vi "setAVGFilterStatus.vi"(8 "error in (no error)":errorcluster, 9 "Measurement Function (0: Current)":T2, 10 "AVG Filter type":T1, 11 "Electrometer in":refnum<class "Electrometer.lvclass">) -> (0 "error out":errorcluster, 3 "Electrometer out":refnum<class "Electrometer.lvclass">)   [LabVIEW 2016, in "Electrometer.lvclass"]
uses:
  Electrometer.lvclass
  Modes.ctl
  AVG Filter type.ctl
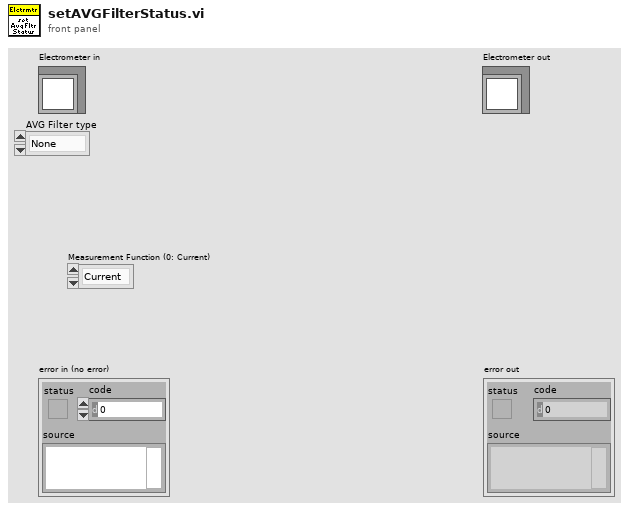
[diagram p1: front panel]
types:
  T1 = typedef "Electrometer.lvclass/AVG Filter type.ctl" = enum16{"None", "Scalar", "Advanced"}
  T2 = typedef "Electrometer.lvclass/Modes.ctl" = enum16{"Current", "Charge", "Voltage", "Resistance"}
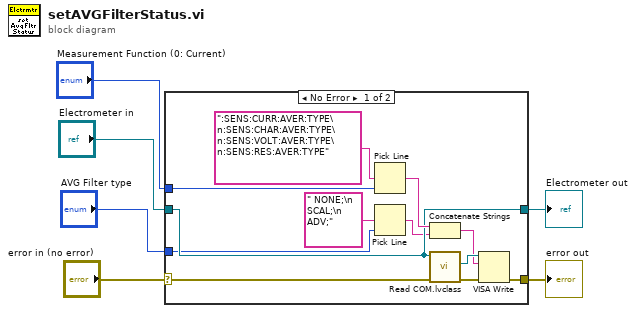
[diagram p0: block diagram]
diagram:
  n1 = case shown="No Error" "error in (no error)" {
    selector: "error in (no error)" -> [w13 w20]
    tunnel: [w11 w20] -> w5
    tunnel: [w14 w19] -> w3
    tunnel: "Electrometer in" -> [w14 w19]
    tunnel: "Measurement Function (0: Current)" -> [w10 _]
    tunnel: "AVG Filter type" -> [w7 _]
    frame No Error {
      n2 = Pick Line(multi-line string=":SENS:CURR:AVER:TYPE\n:SENS:CHAR:AVER:TYPE\n:SENS:VOLT:AVER:TYPE\n:SENS:RES:AVER:TYPE", line index=w10) -> (output string=w15:string)  [unwired: 1 in]
      n3 = Pick Line(multi-line string=" NONE;\n SCAL;\n ADV;", line index=w7) -> (output string=w8:string)  [unwired: 1 in]
      n4 = Concatenate Strings(w15, w8) -> (w17:string)
      n5 = call "Read COM.lvclass.vi"("error in (no error)"=w13, "Electrometer in"=w14) -> ("error out"=w12:errorcluster, "VISA"=w18:refnum<visa-resource-name>)  [unwired: 7 in, 1 out]
      n6 = VISA Write(VISA resource name=w18, write buffer=w17, error in (no error)=w12) -> (error out=w11:errorcluster)  [unwired: 2 out]
    }
    frame Error {
    }
  }
  "error out" <- w5
  "Electrometer out" <- w3
